vi "Climb.vi"(7 "Description":string, 8 "Command Info In":T1, 9 "Vision Tracking":bool, 11 "Driver Stick Y":dbl) -> (0 "Command Info Out":T1)   [LabVIEW 2017]
uses:
  <vilib>/Rock Robotics/WPI/Framework/Command Status Info.ctl
  <vilib>/Rock Robotics/WPI/Framework/Completion Status.ctl
  <vilib>/Rock Robotics/WPI/Framework/Completion Notifier.ctl
  Implementation/Climber Setpoints.ctl
  Implementation/Climber Operations.ctl
panel:
  in  "Duration":dbl
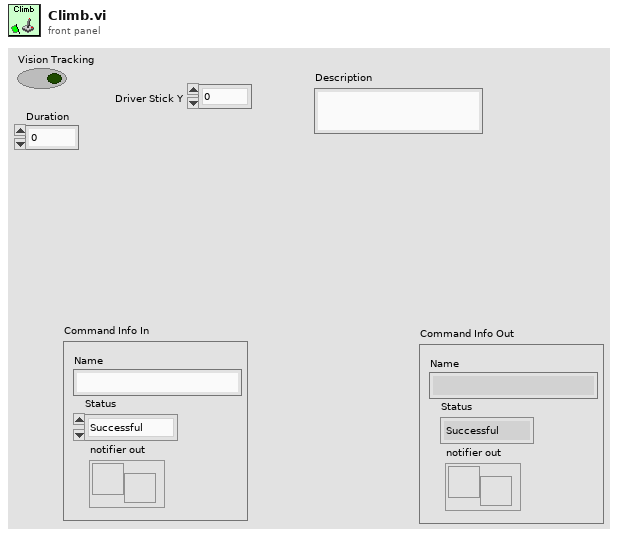
[diagram p1: front panel]
types:
  T1 = typedef "Command Status Info.ctl" = cluster{"Name":string, "Status":T2, "notifier out":T3}
  T2 = typedef "Completion Status.ctl" = enum16{"Successful", "Aborted", "Incomplete"}
  T3 = typedef "Completion Notifier.ctl" = refnum<notifier>
  T4 = typedef "Climber Setpoints.ctl" = cluster{"Operation":T5, "Climber Speed":dbl, "Duration":dbl, "X":dbl, "X 2":dbl, "Vision Tracking":bool}
  T5 = typedef "Climber Operations.ctl" = enum16{"Reserve", "Read Current", "Climb"}
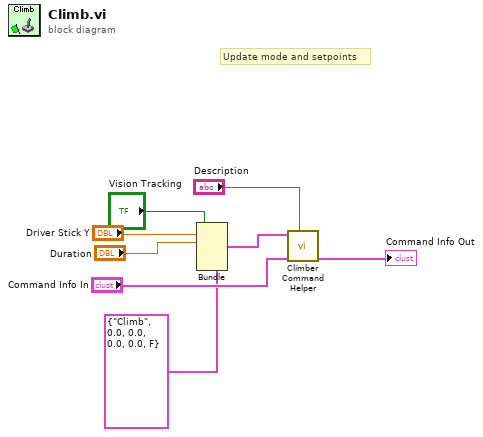
[diagram p0: block diagram]
diagram:
  # "Update mode and setpoints"
  n1 = Bundle(cluster=T4 {"Operation"=enum."Climb", "Climber Speed"=0.0, "Duration"=0.0, "X"=0.0, "X 2"=0.0, "Vision Tracking"=FALSE} ("SubSystem Data"), "Climber Speed"="Driver Stick Y", "Duration"="Duration", "Vision Tracking"="Vision Tracking") -> (w3:T4)  [unwired: 3 in]
  n2 = call "Climber Command Helper.vi"("Description"="Description", "Command Info In"="Command Info In", "SubSystem Data"=w3) -> ("Command Info Out"=→"Command Info Out":T1)  [unwired: 7 in, 1 out]
